vi "Get Event Data In.vi"(8 "error in (no error)":errorcluster, 10 "Event Data Names":string[](array[string]), 11 "Diagram in":refnum<vi>) -> (0 "error out":errorcluster, 2 "OutputTerms[]":refnum<vi>[](array[refnum]), 3 "Diagram out":refnum<vi>)   [LabVIEW 2015, in "Scripting.lvlib"]
uses:
  Scripting.lvlib
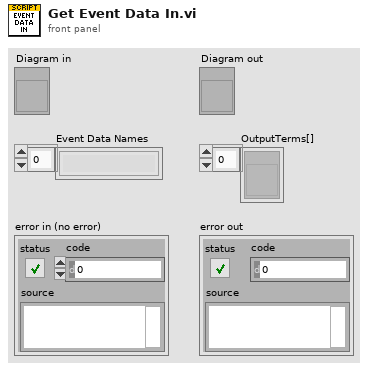
[diagram p1: front panel]
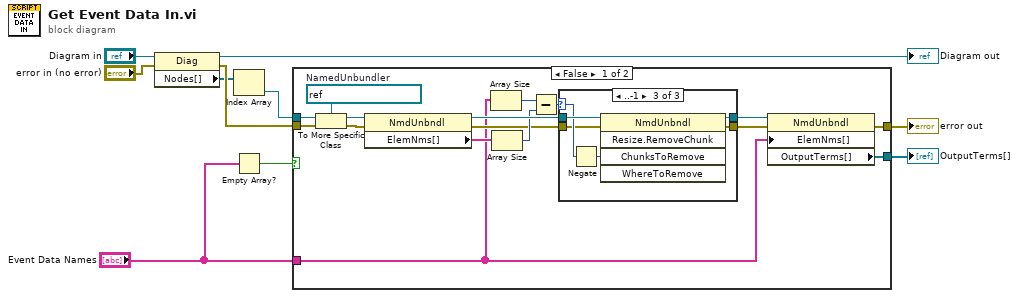
[diagram p0: block diagram]
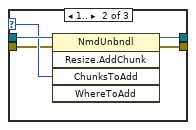
[diagram p3: hidden frame]
diagram:
  n1 = property class="Diag"(reference="Diagram in", error in="error in (no error)") -> (reference out=→"Diagram out":refnum<vi>, error out=w6:errorcluster, "Nodes[]"=w4:refnum<vi>[])
  n2 = Index Array(array=w4) -> (element=w5:refnum<vi>)  [unwired: 1 in]
  n3 = Empty Array?(array="Event Data Names") -> (empty?=w8:bool)
  n4 = case shown="False" w8 {
    tunnel: w5 -> [w26 _]
    tunnel: w6 -> [w25 w40]
    tunnel: "Event Data Names" -> [w11 _]
    tunnel: [w18 w40] -> w10
    tunnel: [w19 _] -> w9
    frame False {
      w24 = refnum<vi> refnum  # NamedUnbundler
      n5 = To More Specific Class(target class=w24, reference=w26, error in=w25) -> (specific class reference=w16:refnum<vi>, error out=w13:errorcluster)
      n6 = property class="NmdUnbndl"(reference=w16, error in=w13) -> (reference out=w23:refnum<vi>, error out=w12:errorcluster, "ElemNms[]"=w22:string[])
      n7 = Array Size(array=w11) -> (size(s)=w20:i32)
      n8 = Array Size(array=w22) -> (size(s)=w21:i32)
      n9 = Subtract(x=w20, y=w21) -> (x-y=w17:i32)
      n10 = case shown="..-1" w17 {
        selector: w17 -> [_ w32 w38]
        tunnel: w23 -> [w28 w33 w39]
        tunnel: [w28 w31 w37] -> w15
        tunnel: w12 -> [w27 w30 w35]
        tunnel: [w27 w29 w36] -> w14
        frame 0 {
        }
        frame 1.. {
          n11 = invoke class="NmdUnbndl" method="Resize.AddChunk"(reference=w33, error in=w30, "ChunksToAdd"=w32) -> (reference out=w31:refnum<vi>, error out=w29:errorcluster)  [unwired: 2 in, 3 out]
        }
        frame ..-1 {
          n12 = Negate(x=w38) -> (-x=w34:i32)
          n13 = invoke class="NmdUnbndl" method="Resize.RemoveChunk"(reference=w39, error in=w35, "ChunksToRemove"=w34) -> (reference out=w37:refnum<vi>, error out=w36:errorcluster)  [unwired: 2 in, 3 out]
        }
      }
      n14 = property class="NmdUnbndl"(reference=w15, error in=w14, "ElemNms[]"=w11) -> (error out=w18:errorcluster, "OutputTerms[]"=w19:refnum<vi>[])  [unwired: 1 out]
    }
    frame True {
    }
  }
  "error out" <- w10
  "OutputTerms[]" <- w9
